vi "GlobalMFCread.vi"() -> ()   [LabVIEW 2013]
panel:
  out "Array":dbl[](array[numeric])
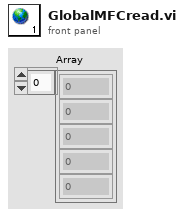
[diagram p1: front panel]
diagram:
